vi "TEMOCR-Initialize Display.vi"(0 "Run":i32, 7 "State":T3, 9 "Total steps":i32, 11 "error in (no error)":errorcluster, 12 "Analysis":T1, 13 "controls":T2) -> (15 "error out":errorcluster)   [LabVIEW 2015]
uses:
  Typedefs/TEMOCR-Analysis State.ctl
  Typedefs/TEMOCR-Controls.ctl
  Typedefs/TEMOCR-Analysis.ctl
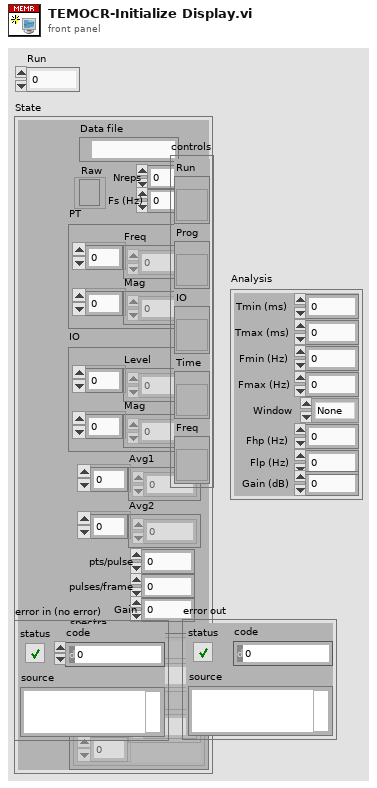
[diagram p1: front panel]
types:
  T1 = typedef "TEMOCR-Analysis.ctl" = cluster{"Tmin (ms)":dbl, "Tmax (ms)":dbl, "Fmin (Hz)":dbl, "Fmax (Hz)":dbl, "Window":enum16{"None", "Hanning", "Hamming"}, "Fhp (Hz)":dbl, "Flp (Hz)":dbl, "Gain (dB)":dbl}
  T2 = typedef "TEMOCR-Controls.ctl" = cluster{"Run":refnum<vi>, "Prog":refnum<vi>, "IO":refnum<vi>, "Time":refnum<vi>, "Freq":refnum<vi>}
  T3 = typedef "TEMOCR-Analysis State.ctl" = cluster{"Data file":path, "Raw":refnum<file>, "PT":cluster{"Freq":dbl[], "Mag":dbl[]}, "IO":cluster{"Level":dbl[], "Mag":dbl[]}, "Nreps":i32, "Fs (Hz)":dbl, "Avg1":dbl[], "pts/pulse":i32, "pulses/frame":i32, "Avg2":dbl[], "Gain":dbl, "spectra":cluster{"Freq":dbl[], "Mag":dbl[][]}[]}
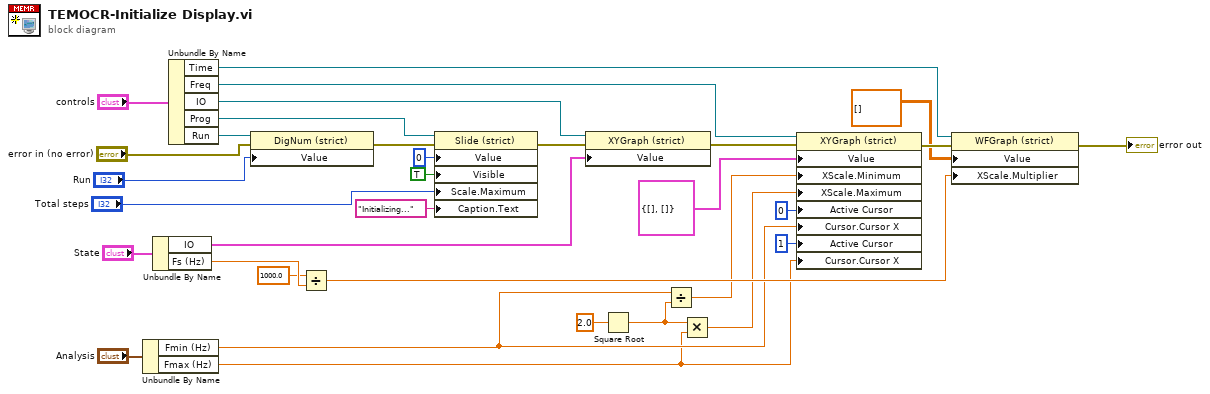
[diagram p0: block diagram]
diagram:
  n1 = Unbundle By Name("Analysis") -> ("Fmin (Hz)"=w5:dbl, "Fmax (Hz)"=w3:dbl)
  n2 = Unbundle By Name("State") -> ("IO"=w22:cluster{"Level":dbl[], "Mag":dbl[]}, "Fs (Hz)"=w13:dbl)
  n3 = Unbundle By Name("controls") -> ("Time"=w18:refnum<vi>, "Freq"=w21:refnum<vi>, "IO"=w25:refnum<vi>, "Prog"=w30:refnum<vi>, "Run"=w32:refnum<vi>)
  n4 = property class="DigNum (strict)"(reference=w32, error in="error in (no error)", "Value"="Run") -> (error out=w29:errorcluster)  [unwired: 1 out]
  n5 = Divide(x=1000.0, y=w13) -> (x/y=w11:dbl)
  n6 = property class="Slide (strict)"(reference=w30, error in=w29, "Value"=u8 0, "Visible"=TRUE, "Scale.Maximum"="Total steps", "Caption.Text"="Initializing...") -> (error out=w24:errorcluster)  [unwired: 1 out]
  n7 = property class="XYGraph (strict)"(reference=w25, error in=w24, "Value"=w22) -> (error out=w20:errorcluster)  [unwired: 1 out]
  n8 = Square Root(x=2.0) -> (sqrt(x)=w7:dbl)
  n9 = Divide(x=w5, y=w7) -> (x/y=w10:dbl)
  n10 = Multiply(x=w7, y=w3) -> (x*y=w8:dbl)
  n11 = property class="XYGraph (strict)"(reference=w21, error in=w20, "Value"=cluster{dbl[], dbl[]} {[], []}, "XScale.Minimum"=w10, "XScale.Maximum"=w8, "Active Cursor"=u32 0, "Cursor.Cursor X"=w5, "Active Cursor"=u32 1, "Cursor.Cursor X"=w3) -> (error out=w17:errorcluster)  [unwired: 1 out]
  n12 = property class="WFGraph (strict)"(reference=w18, error in=w17, "Value"=dbl[][] [], "XScale.Multiplier"=w11) -> (error out=→"error out":errorcluster)  [unwired: 1 out]
